vi "Input_Beam_Check_Locations.vi"() -> ()   [LabVIEW 2020]
uses:
  Globals/Constants_global.vi
  Gen Trav/Trav_mode.ctl
  Controls/User_Specific_mode.ctl
  Controls/Tunnel_Coordinates.ctl
  File/Setup_Filetype.ctl
  Globals/LDA_global.vi
panel:
  out "Channel":i32
  out "Setup group":string[][](array[string])
  out "All Beams":bool
  out "BSA IP":string
  out "Unshifted":bool
  out "Laser IP":string
  out "Beam Info":T1(array[cluster])
  in  "Mode":T2(ring)
  out "setups":string[](array[string])
  in  "Traverse Control":T3(array[cluster]) {"Position Change" format="%#.2f"; "Current Position" format="%#.2f"}
  out "Beams to check":string[](array[string])
  out "Error Message":string
  in  "stop":bool
  out "Results":string[][](table)
  out "Working On":string="Green Shifted"
  in  "OK Button":bool
  out "Message":string
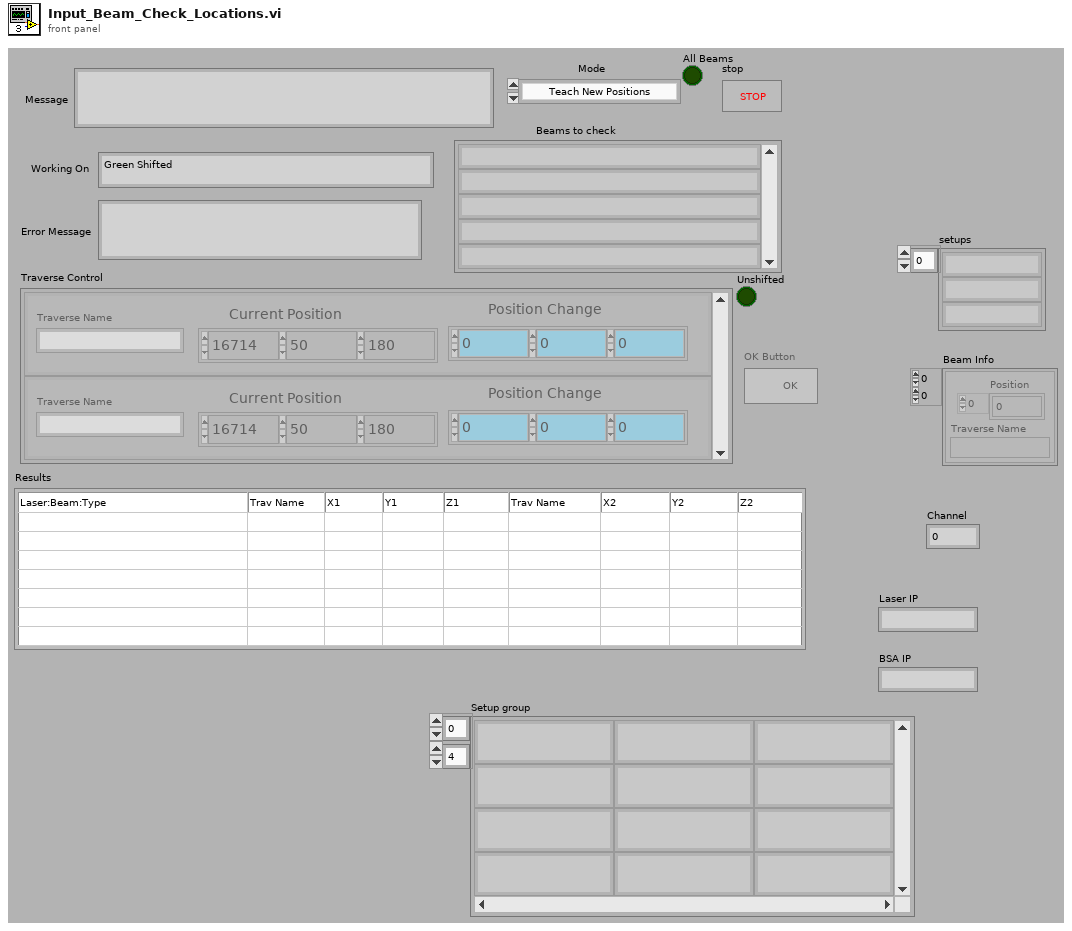
[diagram p1: front panel]
types:
  T1 = cluster{"Position":sgl[], "Traverse Name":string}[][]
  T2 = enum16{"Teach New Positions", "Update Existing Positions"}
  T3 = cluster{"Traverse Name":string, "Current Position":sgl[], "Position Change":sgl[]}[]
  T4 = enum16{"Zero or one", "One", "Zero or more", "One or more"}
  T5 = typedef "Setup_Filetype.ctl" = enum16{"Measurement Setups", "Calibration Setups", "General", "Results File Plotter Setups", "Speed Calib Tweaks"}
  T6 = cluster{"Traverse Name":string, "Current Position":sgl[], "Position Change":sgl[]}
  T7 = typedef "Tunnel_Coordinates.ctl" = enum16{"Work in Tunnel Coordinates", "Work in Model Coordinates"}
  T8 = typedef "User_Specific_mode.ctl" = enum16{"Check VI only", "Run VI"}
  T9 = typedef "Trav_mode.ctl" = enum16{"Move traverse", "Read traverse position", "Teach Position"}
  T10 = enum8{"Enabled", "Disabled", "Disabled and Grayed Out"}
  T11 = typedef "LDA_Channel.ctl" = cluster{"Wavelength (nm)":dbl, "Vel Comp":string, "Max Velocity":dbl, "Min Velocity":dbl, "Max Record length":u16, "Signal gain (dB)":i16, "High voltage":i16, "Optics Conversion Factor":dbl, "Min Record length":u16, "Multiply Velocity by -1":bool, "Signal to Noise Ratio":string, "Validation Ratio":string, "Probe":string, "Laser":string, "BSA":string, "Lense":string, "Beam Separation (mm)":dbl, "Focal Length (mm)":dbl, "COLOUR":u32, "BSA IP":string, "Velocity Range (m/s)":dbl, "Centre Velocity (m/s)":dbl, "Unshifted mW":dbl, "Shifted mW":dbl, "Bandwidth Hz":dbl, "Req Sampling Rate Hz":dbl, "Ch":i32, "CenterFreq Hz":dbl, "Laser IP":string, "Sync Delay (s)":dbl}
  T12 = cluster{"Position":dbl[], "Traverse Name":string}[][]
  T13 = cluster{"Position":dbl[], "Traverse Name":string}
  T14 = cluster{"Position":sgl[], "Traverse Name":string}[]
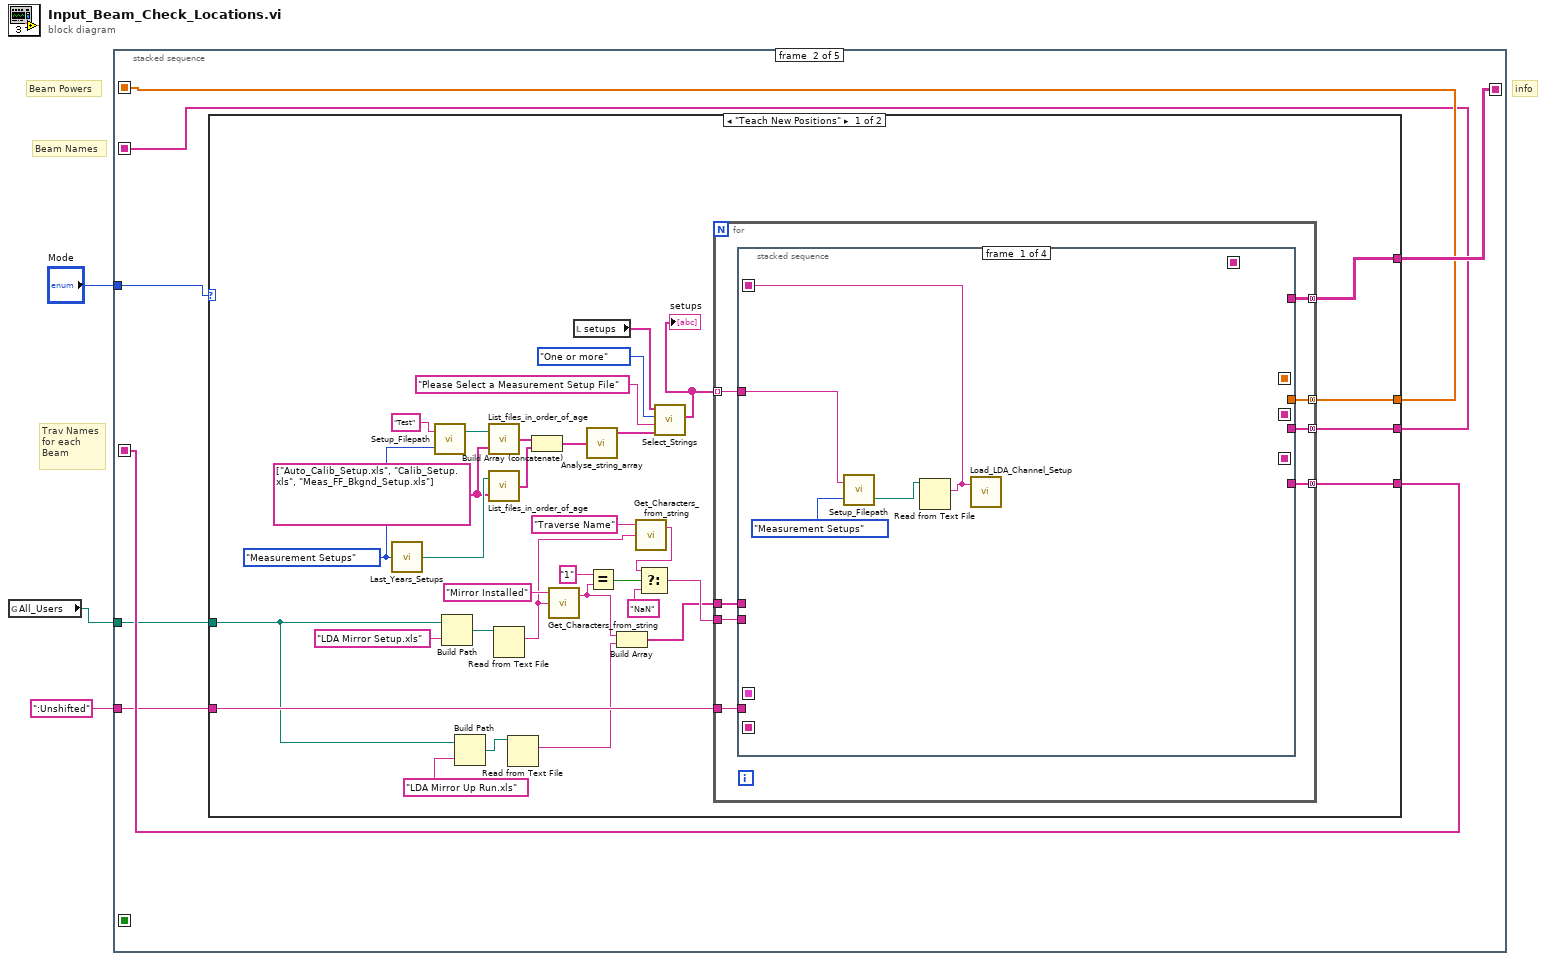
[diagram p0: block diagram]
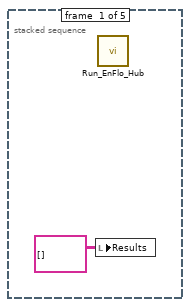
[diagram p2: hidden frame]
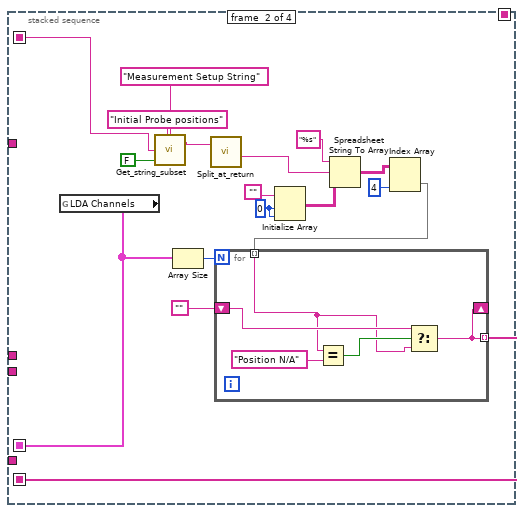
[diagram p3: hidden frame]
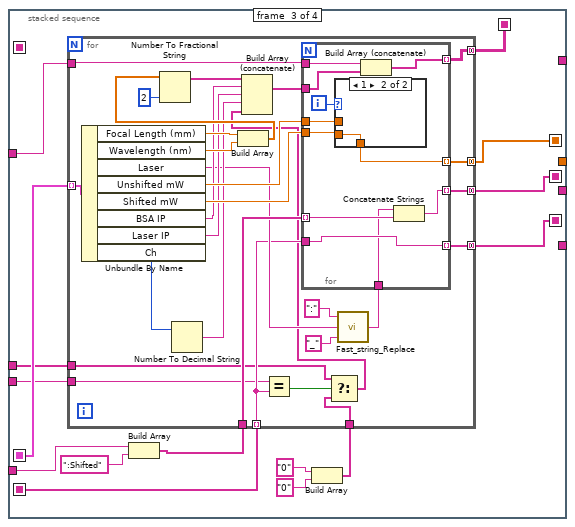
[diagram p4: hidden frame]
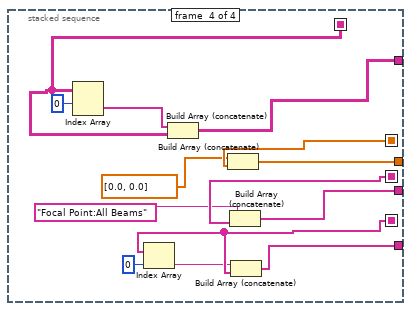
[diagram p6: hidden frame]
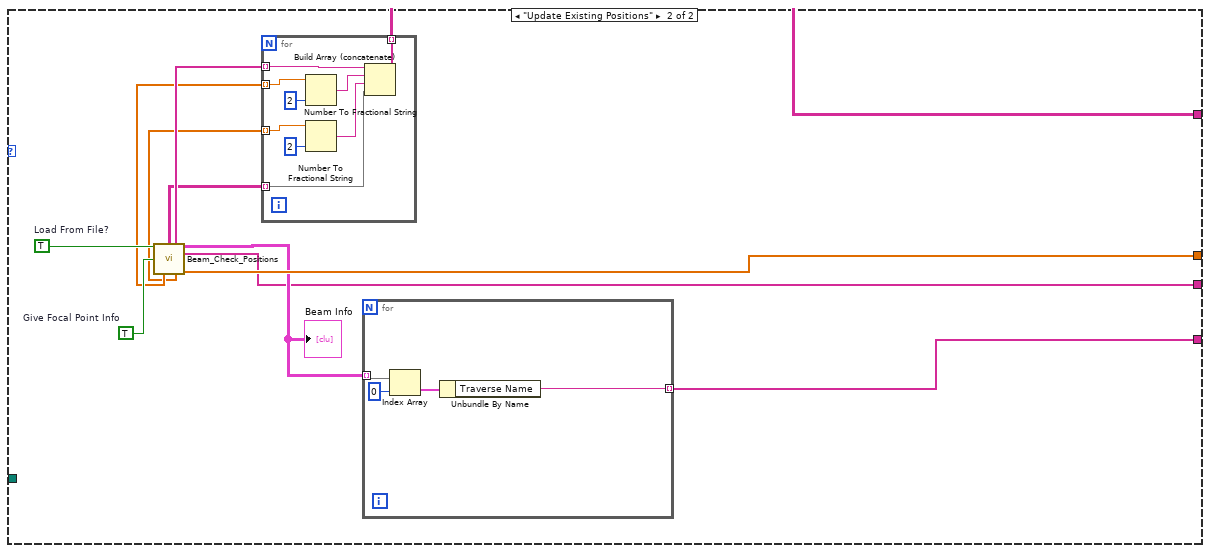
[diagram p7: hidden frame]
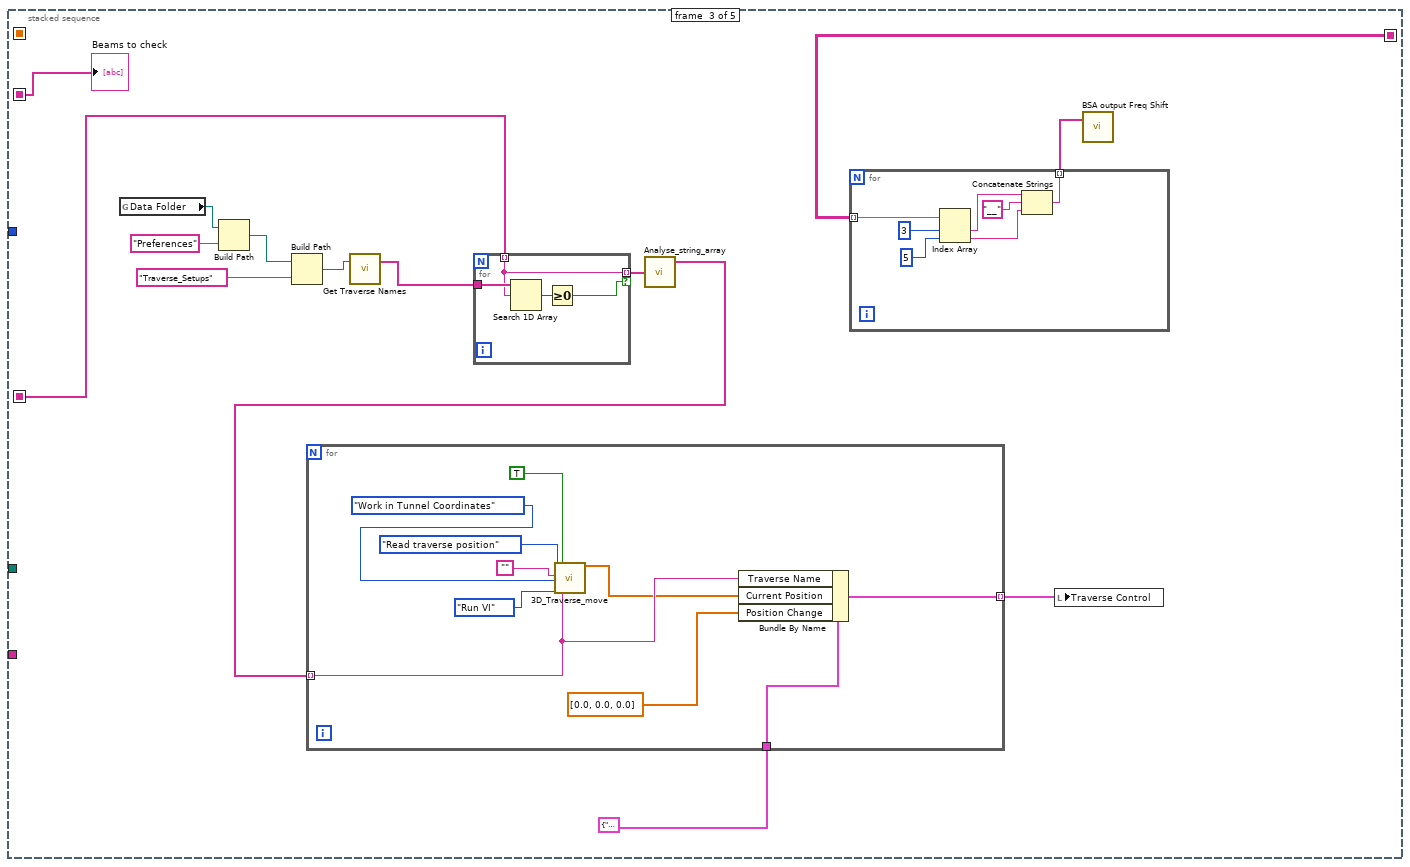
[diagram p8: hidden frame]
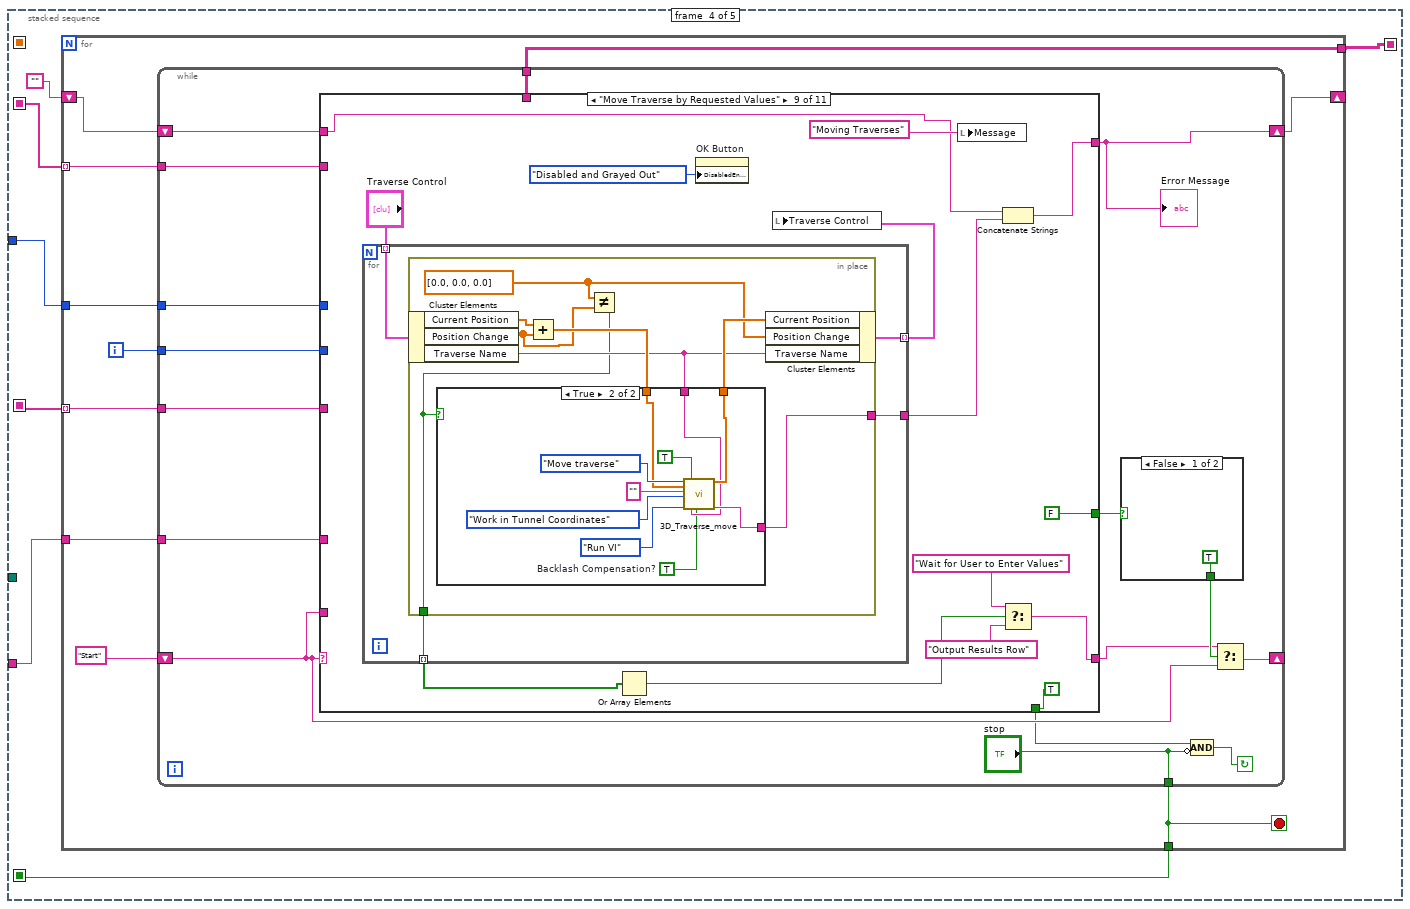
[diagram p9: hidden frame]
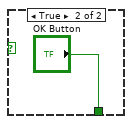
[diagram p10: hidden frame]
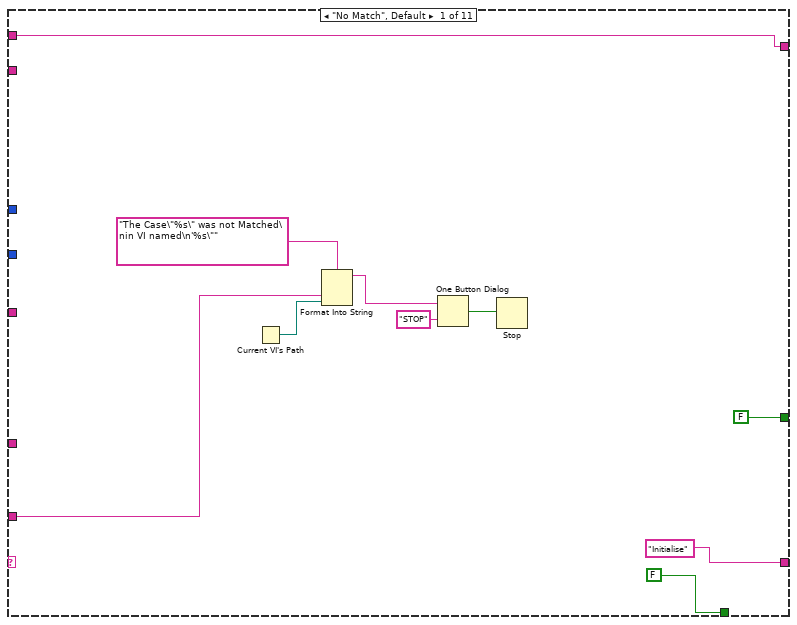
[diagram p11: hidden frame]
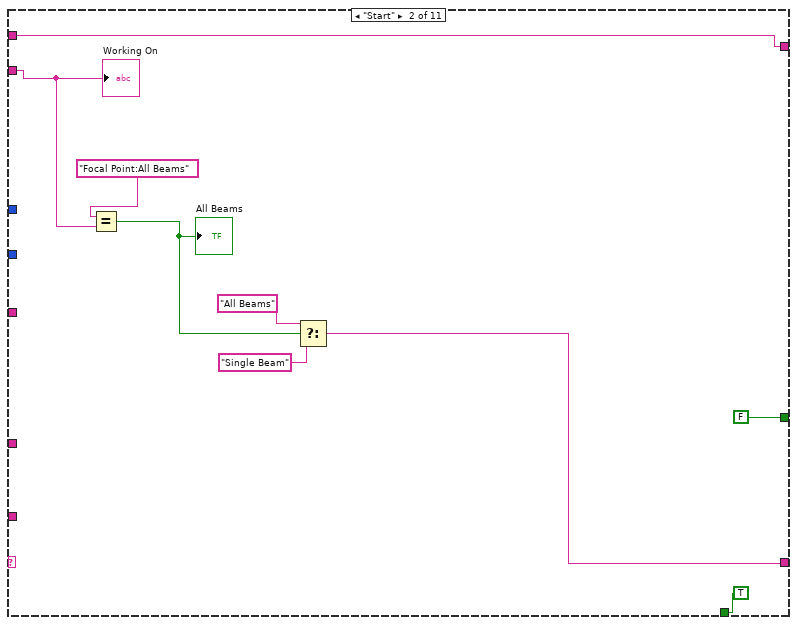
[diagram p12: hidden frame]
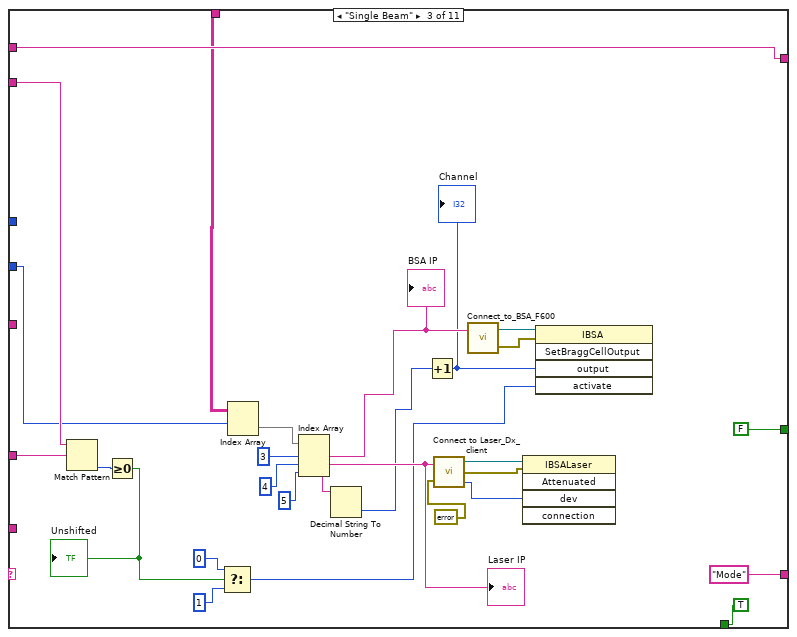
[diagram p13: hidden frame]
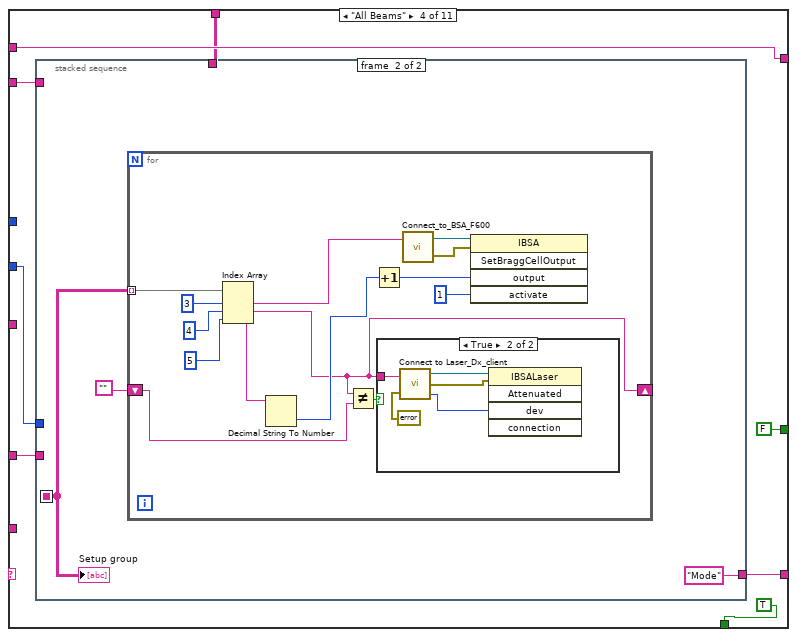
[diagram p14: hidden frame]
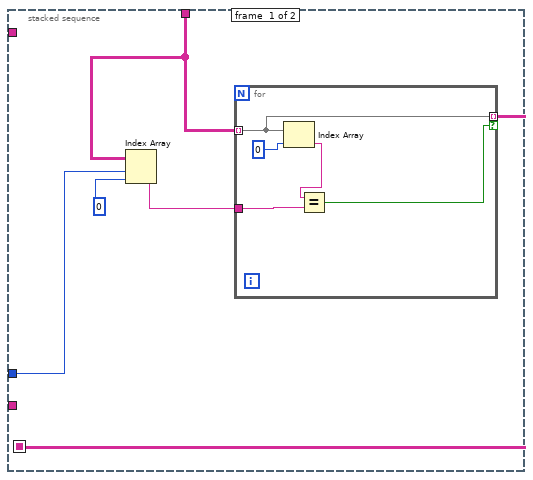
[diagram p15: hidden frame]
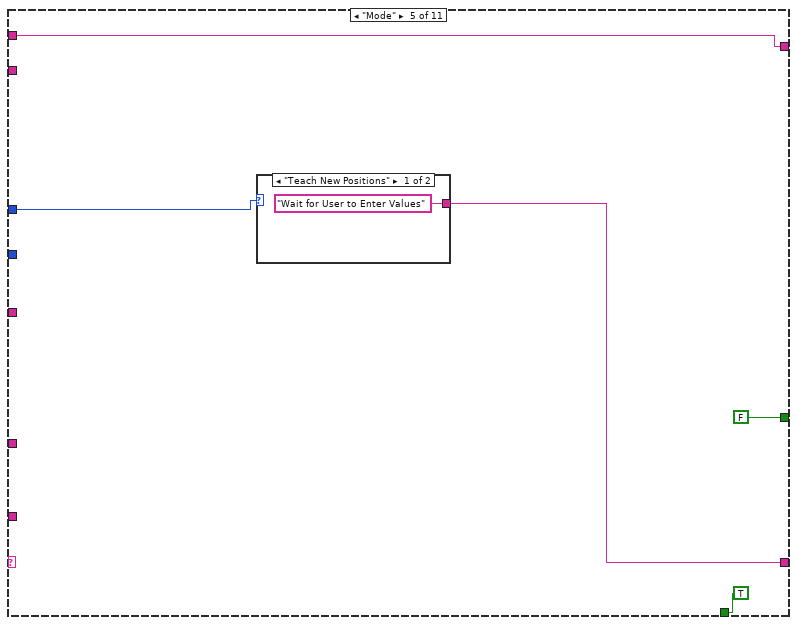
[diagram p17: hidden frame]
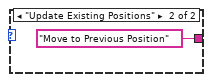
[diagram p18: hidden frame]
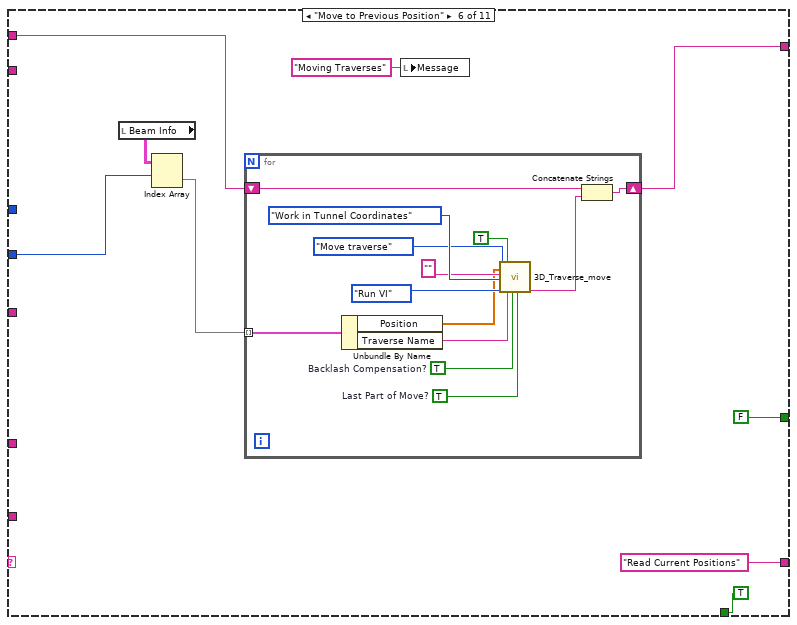
[diagram p19: hidden frame]
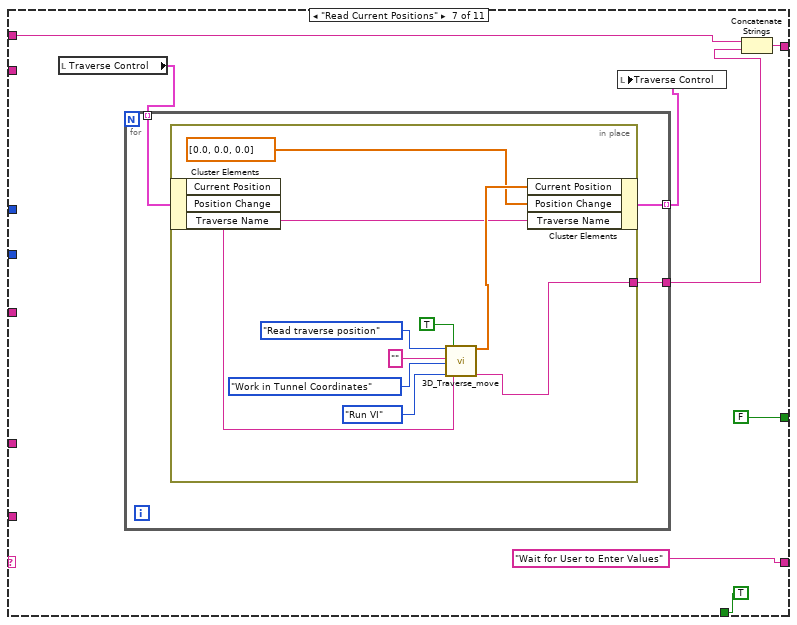
[diagram p20: hidden frame]
diagram:
  # "Beam Powers"
  # "info"
  # "Trav Names\nfor each\nBeam"
  # "Beam Names"
  n1 = global read "Constants_global.vi" "All_Users"() -> (w1:path)
  n2 = stacked-sequence {
    seq-local: [_ w11 _ _ _] -> [_ _ w182 w214 _]
    seq-local: [_ w8 _ _ _] -> [_ _ w179 w216 _]
    seq-local: [_ w10 _ _ _] -> [_ _ w178 w210 w494]
    seq-local: [_ w9 _ _ _] -> [_ _ _ _ w492]
    seq-local: [_ _ _ w213 _] -> [_ _ _ _ w493]
    tunnel: "Mode" -> [_ w7 _ w212 _]
    tunnel: ":Unshifted" ("f") -> [_ w6 _ w211 _]
    tunnel: w1 -> [_ w5 _ _ _]
    frame #0 {
      n3 = local write "Results"(string[][] [] ("Results")) -> ()
      n4 = call "Run_EnFlo_Hub.vi"() -> ()  [unwired: 7 in, 1 out]
    }
    frame #1 {
      n5 = case shown="\"Teach New Positions\"" w7 {
        tunnel: [w33 w158] -> w11
        tunnel: [w32 w155] -> w10
        tunnel: [w31 w160] -> w9
        tunnel: [w30 w157] -> w8
        tunnel: w6 -> [w28 _]
        tunnel: w5 -> [w22 _]
        frame "Teach New Positions" {
          w40 = string[] ["Auto_Calib_Setup.xls", "Calib_Setup.xls", "Meas_FF_Bkgnd_Setup.xls"] ("file names")
          w39 = Setup_Filetype."Measurement Setups" ("Setup File Type")
          n6 = call "Last_Years_Setups.vi"("Setup File Type"=w39) -> ("Directory"=w41:path)
          n7 = call "Setup_Filepath.vi"("Setup File Type"=w39, "Filename in"="Test") -> ("Directory"=w44:path)  [unwired: 1 out]
          n8 = Build Path(base path=w22, name or relative path="LDA Mirror Setup.xls") -> (appended path=w25:path)
          n9 = Build Path(base path=w22, name or relative path="LDA Mirror Up Run.xls") -> (appended path=w23:path)
          n10 = call "List_files_in_order_of_age.vi"("Files to Hide"=w40, "Folder"=w44) -> ("file names"=w38:string[])
          n11 = call "List_files_in_order_of_age.vi"("Files to Hide"=w40, "Folder"=w41) -> ("file names"=w37:string[])
          n12 = Read from Text File(file (use dialog)=w25) -> (text=w17:string)  [unwired: 3 in, 3 out]
          n13 = Read from Text File(file (use dialog)=w23) -> (text=w21:string)  [unwired: 3 in, 3 out]
          n14 = Build Array (concatenate)(w38, w37) -> (w36:string[])
          n15 = call "Get_Characters_from_string.vi"("Input string"=w17, "Variable name"="Mirror Installed") -> ("Value"=w19:string)  [unwired: 1 in, 1 out]
          n16 = local read "setups"() -> (w34:string[])
          n17 = call "Analyse_string_array.vi"("String array"=w36) -> ("Unique strings"=w35:string[])  [unwired: 1 in, 1 out]
          n18 = Equal?(x="1", y=w19) -> (x = y?=w16:bool)
          n19 = Build Array(w19, w21) -> (w12:string[])
          n20 = call "Get_Characters_from_string.vi"("Input string"=w17, "Variable name"="Traverse Name") -> ("Value"=w15:string)  [unwired: 1 in, 1 out]
          n21 = Select(t=w15, s=w16, f="NaN") -> (s? t:f=w13:string)
          n22 = call "Select_Strings.vi"("Available Ch names"=w35, "Message"="Please Select a Measurement Setup File", "Selector mode"=T4."One or more", "Desired Ch names (in)"=w34) -> ("Selected Channel Names"=w29:string[])  [unwired: 2 in, 2 out]
          "setups" <- w29
          n23 = for {
            tunnel: w29 -> [w53] mode=indexing
            tunnel: [w52] -> w30 mode=concatenating
            tunnel: [w51] -> w33 mode=concatenating
            tunnel: [w50] -> w32 mode=concatenating
            tunnel: [w49] -> w31 mode=concatenating
            tunnel: w28 -> [w48]
            tunnel: w13 -> [w47]
            tunnel: w12 -> [w46]
            n24 = stacked-sequence {
              seq-local: [w55 _ _ _] -> [_ w63 _ _]
              seq-local: [_ w60 _ _] -> [_ _ w92 _]
              seq-local: [_ w59 _ _] -> [_ _ w91 _]
              seq-local: [_ _ w89 _] -> [_ _ _ w150]
              seq-local: [_ _ w88 _] -> [_ _ _ w148]
              seq-local: [_ _ w87 _] -> [_ _ _ w146]
              seq-local: [_ _ w86 _] -> [_ _ _ w144]
              tunnel: w53 -> [w54 _ w90 _]
              tunnel: [_ _ _ w145] -> w52
              tunnel: [_ _ _ w143] -> w51
              tunnel: [_ _ _ w149] -> w50
              tunnel: [_ _ _ w147] -> w49
              tunnel: w48 -> [_ _ w85 _]
              tunnel: w47 -> [_ _ w84 _]
              tunnel: w46 -> [_ _ w80 _]
              frame #0 {
                n25 = call "Setup_Filepath.vi"("Setup File Type"=Setup_Filetype."Measurement Setups", "Filename in"=w54) -> ("Filename Out"=w56:path)  [unwired: 1 out]
                n26 = Read from Text File(file (use dialog)=w56) -> (text=w55:string)  [unwired: 3 in, 3 out]
                n27 = call "Load_LDA_Channel_Setup.vi"("Setup file string"=w55) -> ()  [unwired: 2 in]
              }
              frame #1 {
                w72 = 0 ("Dimension Size")
                n28 = global read "LDA_global.vi" "LDA Channels"() -> (w60:T11[])
                n29 = call "Get_string_subset.vi"("String Name"="Measurement Setup String", "Show Dialog?"=FALSE, "String to split"=w63, "File Label"="Initial Probe positions") -> ("Output string"=w74:string)  [unwired: 1 out]
                n30 = Array Size(array=w60) -> (size(s)=w61:i32)
                n31 = call "Split_at_return.vi"("String"=w74) -> ("after substring"=w69:string)  [unwired: 1 in, 3 out]
                n32 = Initialize Array("", w72, w72) -> (w73:string[][])
                n33 = Spreadsheet String To Array(format string="%s", spreadsheet string=w69, array type (2D Dbl)=w73) -> (array=w65:string[][])  [unwired: 1 out]
                n34 = Index Array(array=w65, index (col)=4 ("disabled index (col)")) -> (element=w62:string[])  [unwired: 1 in]
                n35 = for {
                  N: w61 -> [_]
                  tunnel: w62 -> [w76] mode=indexing
                  shift-right: [w75] -> _
                  shift-left: "" -> [w77]
                  tunnel: [w75] -> w59 mode=indexing
                  n36 = Equal?(x=w76, y="Position N/A") -> (x = y?=w78:bool)
                  n37 = Select(t=w77, s=w78, f=w76) -> (s? t:f=w75:string)
                }
              }
              frame #2 {
                n38 = Build Array(w85, ":Shifted") -> (w93:string[])
                n39 = Build Array("0", "0") -> (w81:string[])
                n40 = for {
                  tunnel: w92 -> [w123] mode=indexing
                  tunnel: w93 -> [w122]
                  tunnel: [w121] -> w87 mode=concatenating
                  tunnel: w91 -> [w100] mode=indexing
                  tunnel: [w120] -> w86 mode=concatenating
                  tunnel: [w117] -> w88 mode=concatenating
                  tunnel: [w116] -> w89 mode=concatenating
                  tunnel: w90 -> [w115]
                  tunnel: w84 -> [w99]
                  tunnel: w81 -> [w97]
                  tunnel: w80 -> [w96]
                  n41 = Unbundle By Name(w123) -> ("Focal Length (mm)"=w112:dbl, "Wavelength (nm)"=w113:dbl, "Laser"=w104:string, "Unshifted mW"=w119:dbl, "Shifted mW"=w118:dbl, "BSA IP"=w108:string, "Laser IP"=w107:string, "Ch"=w106:i32)
                  n42 = Number To Decimal String(number=w106) -> (decimal integer string=w105:string)  [unwired: 1 in]
                  n43 = Build Array(w112, w113) -> (w111:dbl[])
                  n44 = Number To Fractional String(number=w111, precision (6)=i16 2) -> (F-format string=w110:string[])  [unwired: 2 in]
                  n45 = Equal?(x=w99, y=w100) -> (x = y?=w98:bool)
                  n46 = Select(t=w96, s=w98, f=w97) -> (s? t:f=w95:string[])
                  n47 = Build Array (concatenate)(w110, w108, w107, w105, w95) -> (w109:string[])
                  n48 = call "Fast_string_Replace.vi"("Replace match with:"="_", "Input String"=w104, "regular expression"=":") -> ("Output String"=w101:string)  [unwired: 1 in, 1 out]
                  n49 = for {
                    tunnel: w122 -> [w134] mode=indexing
                    tunnel: [w131] -> w121 mode=indexing
                    tunnel: w100 -> [w128]
                    tunnel: [w128] -> w120 mode=indexing
                    tunnel: w119 -> [w132]
                    tunnel: w118 -> [w130]
                    tunnel: [w129] -> w117 mode=indexing
                    tunnel: [w125] -> w116 mode=indexing
                    tunnel: w115 -> [w127]
                    tunnel: w109 -> [w126]
                    tunnel: w101 -> [w124]
                    i -> [w133]
                    n50 = case shown="1" w133 {
                      tunnel: [w135 w136] -> w129
                      tunnel: w132 -> [w135 _]
                      tunnel: w130 -> [_ w136]
                      frame 0, Default {
                      }
                      frame 1 {
                      }
                    }
                    n51 = Build Array (concatenate)(w127, w126) -> (w125:string[])
                    n52 = Concatenate Strings(w124, w134) -> (w131:string)
                  }
                }
              }
              frame #3 {
                n53 = Index Array(array=w150, index (row)=0) -> (element=w141:string[])  [unwired: 1 in]
                n54 = Index Array(array=w144, index=0 ("index (row)")) -> (element=w137:string)
                n55 = Build Array (concatenate)(w141, w150) -> (w149:string[][])
                n56 = Build Array (concatenate)(dbl[] [0.0, 0.0], w148) -> (w147:dbl[])
                n57 = Build Array (concatenate)("Focal Point:All Beams", w146) -> (w145:string[])
                n58 = Build Array (concatenate)(w137, w144) -> (w143:string[])
              }
            }
          }
        }
        frame "Update Existing Positions" {
          w154 = TRUE  # Give Focal Point Info
          w161 = TRUE  # Load From File?
          n59 = call "Beam_Check_Positions.vi"("Load From File?"=w161, "Give Focal Point Info (F)"=w154) -> ("More Info"=w151:string[][], "Setup File"=w156:string[], "Beam Info"=w159:T12, "Beam Names"=w157:string[], "Focal Length"=w153:dbl[], "Wavelength (nm)"=w152:dbl[], "Power (mW)"=w160:dbl[])  [unwired: 5 in, 2 out]
          "Beam Info" <- w159
          n60 = for {
            tunnel: w156 -> [w170] mode=indexing
            tunnel: w153 -> [w169] mode=indexing
            tunnel: [w167] -> w155 mode=indexing
            tunnel: w152 -> [w166] mode=indexing
            tunnel: w151 -> [w162] mode=indexing
            n61 = Number To Fractional String(number=w169, precision (6)=i16 2) -> (F-format string=w168:string)  [unwired: 2 in]
            n62 = Number To Fractional String(number=w166, precision (6)=i16 2) -> (F-format string=w165:string)  [unwired: 2 in]
            n63 = Build Array (concatenate)(w170, w168, w165, w162) -> (w167:string[])
          }
          n64 = for {
            tunnel: w159 -> [w174] mode=indexing
            tunnel: [w171] -> w158 mode=indexing
            n65 = Index Array(array=w174, index=0) -> (element=w172:T13)
            n66 = Unbundle By Name(w172) -> ("Traverse Name"=w171:string)
          }
        }
      }
    }
    frame #2 {
      n67 = global read "Constants_global.vi" "Data Folder"() -> (w188:path)
      n68 = Build Path(base path=w188, name or relative path="Preferences") -> (appended path=w187:path)
      n69 = Build Path(base path=w187, name or relative path="Traverse_Setups") -> (appended path=w176:path)
      n70 = call "Get Traverse Names.vi"("Traverse\nSetup\nFolder"=w176) -> ("Traverse Names"=w175:string[])  [unwired: 1 in, 1 out]
      n71 = for {
        tunnel: w175 -> [w209]
        tunnel: w182 -> [w207] mode=indexing
        tunnel: [w207] -> w181 mode=indexing if=w206
        n72 = Search 1D Array(1D array=w209, element=w207) -> (index of element=w208:i32)  [unwired: 1 in]
        n73 = Greater Or Equal To 0?(x=w208) -> (x >= 0?=w206:bool)
      }
      n74 = call "Analyse_string_array.vi"("String array"=w181) -> ("Unique strings"=w180:string[])  [unwired: 1 in, 1 out]
      n75 = for {
        tunnel: w180 -> [w202] mode=indexing
        tunnel: T6 {"Traverse Name"="", "Current Position"=[], "Position Change"=[]} ("Cluster 2") -> [w203]
        tunnel: [w198] -> w183 mode=indexing
        n76 = call "3D_Traverse_move.vi"("Mode"=Trav_mode."Read traverse position", "Extra command String"="", "Work in Tunnel Coordinates"=Tunnel_Coordinates."Work in Tunnel Coordinates", "Simulate/Run"=User_Specific_mode."Run VI", "Route Checking?"=TRUE, "Traverse name"=w202) -> ("Trav Position achieved"=w200:sgl[])  [unwired: 10 in, 3 out]
        n77 = Bundle By Name(cluster=w203, "Traverse Name"=w202, "Current Position"=w200, "Position Change"=sgl[] [0.0, 0.0, 0.0]) -> (w198:T6)
      }
      n78 = for {
        tunnel: w178 -> [w193] mode=indexing
        tunnel: [w191] -> w177 mode=indexing
        n79 = Index Array(array=w193, index #1=3 ("index"), index #2=5 ("index")) -> (element #1=w192:string, element #2=w189:string)
        n80 = Concatenate Strings(w192, "__" ("string"), w189) -> (w191:string)
      }
      n81 = local write "Traverse Control"(w183) -> ()
      n82 = call "BSA output Freq Shift.vi"("BSAIP__ChNum"=w177) -> ()  [unwired: 2 in, 1 out]
      "Beams to check" <- w179
    }
    frame #3 {
      n83 = for {
        tunnel: w216 -> [w225] mode=indexing
        shift-right: [w223] -> _
        shift-left: "" -> [w224]
        tunnel: w214 -> [w222] mode=indexing
        tunnel: [w221] -> w213
        tunnel: w212 -> [w220]
        tunnel: w211 -> [w218]
        tunnel: w210 -> [w217]
        i -> [w219]
        stop <- w221 stop-if-true
        n84 = while {
          shift-left: "Start" -> [w240]
          shift-right: [w239] -> _
          shift-right: [w235] -> w223
          shift-left: w224 -> [w234]
          tunnel: w225 -> [w233]
          tunnel: w222 -> [w232]
          tunnel: ["stop"] -> w221
          tunnel: w220 -> [w230]
          tunnel: w219 -> [w229]
          tunnel: w218 -> [w228]
          tunnel: w217 -> [w227]
          stop <- w236 continue-if-true
          n85 = case shown="\"Move Traverse by Requested Values\"" w240 {
            tunnel: [FALSE TRUE TRUE TRUE TRUE TRUE TRUE TRUE TRUE TRUE FALSE] -> w237
            tunnel: ["Initialise" w259 "Mode" ("t") w292 w335 "Read Current Positions" ("t") "Wait for User to Enter Values" ("f") "Move Traverse by Requested Values" w400 "End" ("t") "End" ("t")] -> w241
            tunnel: w240 -> [w249 _ _ _ _ _ _ _ _ _ _]
            tunnel: [FALSE FALSE FALSE FALSE FALSE FALSE FALSE TRUE FALSE FALSE FALSE] -> w238
            tunnel: [w245 w256 w289 w297 w332 w342 w365 w383 w397 w434 w457] -> w235
            tunnel: w234 -> [w245 w256 w289 w297 w332 w343 w363 w383 w396 w434 w457]
            tunnel: w233 -> [_ w262 w286 w295 _ _ _ _ _ _ _]
            tunnel: w232 -> [_ _ _ _ _ _ _ _ _ w430 _]
            tunnel: w230 -> [_ _ _ _ w336 _ _ _ _ _ _]
            tunnel: w229 -> [_ _ w284 w293 _ w345 _ _ _ _ _]
            tunnel: w228 -> [_ _ w288 w296 _ _ _ _ _ _ _]
            tunnel: w227 -> [_ _ w285 w294 _ _ _ _ _ _ _]
            frame "No Match", Default {
              n86 = Current VI's Path() -> (path=w248:path)
              n87 = Format Into String(format string="The Case\"%s\" was not Matched\nin VI named\n'%s\"" ("Format String"), w249, w248) -> (resulting string=w252:string)  [unwired: 2 in, 1 out]
              n88 = One Button Dialog(message=w252, button name ("OK")="STOP") -> (true=w250:bool)
              n89 = Stop(stop? (T)=w250) -> ()
            }
            frame "Start" {
              n90 = Equal?(x="Focal Point:All Beams", y=w262) -> (x = y?=w261:bool)
              "All Beams" <- w261
              n91 = Select(t="All Beams", s=w261, f="Single Beam") -> (s? t:f=w259:string)
              "Working On" <- w262
            }
            frame "Single Beam" {
              n92 = Match Pattern(string=w286, regular expression=w288) -> (offset past match=w287:i32)  [unwired: 1 in, 3 out]
              n93 = Greater Or Equal To 0?(x=w287) -> (x >= 0?=w276:bool)
              "Unshifted" <- w276
              n94 = Select(t=0 ("SetBraggCellOutputFreq"), s=w276, f=1 ("SetBraggCellOutputFreq")) -> (s? t:f=w273:i32)
              n95 = Index Array(array=w285, index (row)=w284) -> (element=w270:string[])  [unwired: 1 in]
              n96 = Index Array(array=w270, index #1=3 ("index"), index #2=4 ("index"), index #3=5 ("index")) -> (element #1=w277:string, element #2=w283:string, element #3=w266:string)
              "Laser IP" <- w283
              "BSA IP" <- w277
              n97 = Decimal String To Number(string=w266) -> (number=w272:i32)  [unwired: 2 in, 1 out]
              n98 = Increment(x=w272) -> (x+1=w265:i32)
              "Channel" <- w265
              n99 = call "Connect to Laser_Dx_client.vi"("Laser IP Number"=w283, "error in (no error)"=errorcluster {"status"=FALSE, "code"=0, "source"=""}) -> ("Laser_Dx"=w282:refnum<k7>, "error out"=w281:errorcluster, "Channel"=w280:i64)
              n100 = call "Connect_to_BSA_F600.vi"("BSA IP Number"=w277) -> ("error out"=w278:errorcluster, "F600"=w279:refnum<k7>)  [unwired: 1 in]
              n101 = invoke class="IBSALaser" method="Attenuated"(reference=w282, error in=w281, "dev"=w280) -> ()  [unwired: 2 in, 5 out]
              n102 = invoke class="IBSA" method="SetBraggCellOutput"(reference=w279, error in=w278, "output"=w265, "activate"=w273) -> ()  [unwired: 1 in, 5 out]
            }
            frame "All Beams" {
              n103 = stacked-sequence {
                seq-local: [w300 _] -> [_ w311]
                tunnel: w296 -> [_ _]
                tunnel: w295 -> [_ _]
                tunnel: w294 -> [w301 _]
                tunnel: w293 -> [w304 _]
                tunnel: [_ "Mode" ("t")] -> w292
                frame #0 {
                  n104 = Index Array(array=w301, index (row)=w304, index (col)=0 ("disabled index (col)")) -> (element=w302:string)
                  n105 = for {
                    tunnel: w302 -> [w309]
                    tunnel: w301 -> [w306] mode=indexing
                    tunnel: [w306] -> w300 mode=indexing if=w305
                    n106 = Index Array(array=w306, index=0 ("disabled index (col)")) -> (element=w307:string)
                    n107 = Equal?(x=w307, y=w309) -> (x = y?=w305:bool)
                  }
                }
                frame #1 {
                  n108 = for {
                    shift-right: [w316] -> _
                    shift-left: "" -> [w315]
                    tunnel: w311 -> [w317] mode=indexing
                    n109 = Index Array(array=w317, index #1=3 ("index"), index #2=4 ("index"), index #3=5 ("index")) -> (element #1=w324:string, element #2=w316:string, element #3=w319:string)
                    n110 = Decimal String To Number(string=w319) -> (number=w323:i32)  [unwired: 2 in, 1 out]
                    n111 = Not Equal?(x=w316, y=w315) -> (x != y?=w314:bool)
                    n112 = Increment(x=w323) -> (x+1=w313:i32)
                    n113 = case shown="True" w314 {
                      tunnel: w316 -> [_ w331]
                      frame False {
                      }
                      frame True {
                        n114 = call "Connect to Laser_Dx_client.vi"("Laser IP Number"=w331, "error in (no error)"=errorcluster {"status"=FALSE, "code"=0, "source"=""}) -> ("Laser_Dx"=w330:refnum<k7>, "error out"=w329:errorcluster, "Channel"=w328:i64)
                        n115 = invoke class="IBSALaser" method="Attenuated"(reference=w330, error in=w329, "dev"=w328) -> ()  [unwired: 2 in, 5 out]
                      }
                    }
                    n116 = call "Connect_to_BSA_F600.vi"("BSA IP Number"=w324) -> ("error out"=w325:errorcluster, "F600"=w326:refnum<k7>)  [unwired: 1 in]
                    n117 = invoke class="IBSA" method="SetBraggCellOutput"(reference=w326, error in=w325, "output"=w313, "activate"=1 ("SetBraggCellOutputFreq")) -> ()  [unwired: 1 in, 5 out]
                  }
                  "Setup group" <- w311
                }
              }
            }
            frame "Mode" {
              n118 = case shown="\"Teach New Positions\"" w336 {
                tunnel: ["Wait for User to Enter Values" ("f") "Move to Previous Position"] -> w335
                frame "Teach New Positions" {
                }
                frame "Update Existing Positions" {
                }
              }
            }
            frame "Move to Previous Position" {
              n119 = local read "Beam Info"() -> (w347:T1)
              n120 = Index Array(array=w347, index (row)=w345) -> (element=w346:T14)  [unwired: 1 in]
              n121 = for {
                shift-right: [w353] -> w342
                shift-left: w343 -> [w352]
                tunnel: w346 -> [w350] mode=indexing
                w348 = TRUE  # Last Part of Move?
                w349 = TRUE  # Backlash Compensation?
                n122 = Unbundle By Name(w350) -> ("Position"=w355:sgl[], "Traverse Name"=w354:string)
                n123 = call "3D_Traverse_move.vi"("Mode"=Trav_mode."Move traverse", "Position"=w355, "Extra command String"="", "Work in Tunnel Coordinates"=Tunnel_Coordinates."Work in Tunnel Coordinates", "Simulate/Run"=User_Specific_mode."Run VI", "Route Checking?"=TRUE, "Traverse name"=w354, "Backlash Compensation?"=w349, "Last Part of Move?"=w348) -> ("Error String"=w351:string)  [unwired: 7 in, 3 out]
                n124 = Concatenate Strings(w352, w351) -> (w353:string)
              }
              n125 = local write "Message"("Moving Traverses" ("Message")) -> ()
            }
            frame "Read Current Positions" {
              n126 = local read "Traverse Control"() -> (w368:T3)
              n127 = for {
                tunnel: [w371] -> w364
                tunnel: w368 -> [w370] mode=indexing
                tunnel: [w369] -> w366 mode=indexing
                n128 = in-place {
                  in-place-border: [w380] -> w371
                  n129 = in-place-cluster #1(w370) -> ("Traverse Name"=w377:string)  [unwired: 2 out]
                  n130 = call "3D_Traverse_move.vi"("Mode"=Trav_mode."Read traverse position", "Extra command String"="", "Work in Tunnel Coordinates"=Tunnel_Coordinates."Work in Tunnel Coordinates", "Simulate/Run"=User_Specific_mode."Run VI", "Route Checking?"=TRUE, "Traverse name"=w377) -> ("Trav Position achieved"=w379:sgl[], "Error String"=w380:string)  [unwired: 10 in, 2 out]
                  n131 = in-place-cluster #1("Current Position"=w379, "Position Change"=sgl[] [0.0, 0.0, 0.0] ("Green Position Change"), "Traverse Name"=w377) -> (w369:T6)
                }
              }
              n132 = local write "Traverse Control"(w366) -> ()
              n133 = Concatenate Strings(w363, w364) -> (w365:string)
            }
            frame "Wait for User to Enter Values" {
              n134 = local read "Working On"() -> (w384:string)
              n135 = property on="OK Button" class="Bool"("DisabledEnum"=T10."Enabled" ("Disabled")) -> ()  [unwired: 2 in, 2 out]
              n136 = Format Into String(format string="Please get the %s beam into the power meter by editing Positions then Press OK", w384) -> (resulting string=→"Message":string)  [unwired: 2 in, 1 out]
            }
            frame "Move Traverse by Requested Values" {
              n137 = for {
                tunnel: [w406] -> w398
                tunnel: "Traverse Control" -> [w405] mode=indexing
                tunnel: [w404] -> w394 mode=indexing
                tunnel: [w403] -> w391 mode=indexing
                n138 = in-place {
                  in-place-border: [w414] -> w406
                  in-place-border: [w407] -> w404
                  w409 = sgl[] [0.0, 0.0, 0.0] ("Green Position Change")
                  n139 = in-place-cluster #2(w405) -> ("Current Position"=w413:sgl[], "Position Change"=w410:sgl[], "Traverse Name"=w408:string)
                  n140 = Add(x=w413, y=w410) -> (x+y=w412:sgl[])
                  n141 = Not Equal?(x=w409, y=w410) -> (x != y?=w407:bool)
                  n142 = case shown="True" w407 {
                    tunnel: ["" w426] -> w414
                    tunnel: w412 -> [w416 w420]
                    tunnel: [w416 w419] -> w411
                    tunnel: w408 -> [_ w418]
                    frame False {
                    }
                    frame True {
                      w417 = TRUE  # Backlash Compensation?
                      n143 = call "3D_Traverse_move.vi"("Mode"=Trav_mode."Move traverse", "Position"=w420, "Extra command String"="", "Work in Tunnel Coordinates"=Tunnel_Coordinates."Work in Tunnel Coordinates", "Simulate/Run"=User_Specific_mode."Run VI", "Route Checking?"=TRUE, "Traverse name"=w418, "Backlash Compensation?"=w417) -> ("Trav Position achieved"=w419:sgl[], "Error String"=w426:string)  [unwired: 8 in, 2 out]
                    }
                  }
                  n144 = in-place-cluster #2("Current Position"=w411, "Position Change"=w409, "Traverse Name"=w408) -> (w403:T6)
                }
              }
              n145 = Or Array Elements(Boolean array=w394) -> (logical OR=w393:bool)
              n146 = property on="OK Button" class="Bool"("DisabledEnum"=T10."Disabled and Grayed Out" ("Disabled")) -> ()  [unwired: 2 in, 2 out]
              n147 = local write "Traverse Control"(w391) -> ()
              n148 = local write "Message"("Moving Traverses") -> ()
              n149 = Concatenate Strings(w396, w398) -> (w397:string)
              n150 = Select(t="Wait for User to Enter Values" ("f"), s=w393, f="Output Results Row" ("t")) -> (s? t:f=w400:string)
            }
            frame "Output Results Row" {
              n151 = local read "Traverse Control"() -> (w429:T3)
              n152 = for {
                tunnel: w429 -> [w449] mode=indexing
                tunnel: [w448] -> w431 mode=indexing
                n153 = Unbundle By Name(w449) -> ("Traverse Name"=w448:string)
              }
              n154 = local read "Working On"() -> (w438:string)
              n155 = Search 1D Array(1D array=w431, element=w430) -> (index of element=w427:i32)  [unwired: 1 in]
              n156 = case shown="Default" w427 {
                selector: w427 -> [w441 _]
                tunnel: w429 -> [w445 w447]
                tunnel: [w442 w447] -> w428
                frame Default {
                  n157 = Delete From Array(array=w445, length=1, index=w441) -> (array with subset deleted=w443:T3)  [unwired: 1 out]
                  n158 = Index Array(array=w445, index=w441) -> (element=w444:T6)
                  n159 = Build Array (concatenate)(w444, w443) -> (w442:T3)
                }
                frame -1 {
                }
              }
              n160 = for {
                tunnel: w428 -> [w455] mode=indexing
                tunnel: [w450] -> w432 mode=concatenating
                n161 = Unbundle By Name(w455) -> ("Traverse Name"=w451:string, "Current Position"=w453:sgl[])
                n162 = Number To Fractional String(number=w453, precision (6)=i16 2) -> (F-format string=w452:string[])  [unwired: 2 in]
                n163 = Build Array (concatenate)(w451, w452) -> (w450:string[])
              }
              n164 = Build Array (concatenate)(w438, w432) -> (w436:string[])
              n165 = local read "Results"() -> (w437:string[][])
              n166 = Build Array (concatenate)(w437, w436) -> (→"Results":string[][])
            }
            frame "End" {
              n167 = local read "All Beams"() -> (w456:bool)
              n168 = case shown="True" w456 {
                frame False {
                  n169 = local read "Laser IP"() -> (w466:string)
                  n170 = local read "BSA IP"() -> (w467:string)
                  n171 = local read "Channel"() -> (w462:i32)
                  n172 = call "Connect to Laser_Dx_client.vi"("Laser IP Number"=w466, "error in (no error)"=errorcluster {"status"=FALSE, "code"=0, "source"=""}) -> ("Laser_Dx"=w465:refnum<k7>, "error out"=w464:errorcluster, "Channel"=w463:i64)
                  n173 = call "Connect_to_BSA_F600.vi"("BSA IP Number"=w467) -> ("error out"=w469:errorcluster, "F600"=w470:refnum<k7>)  [unwired: 1 in]
                  n174 = invoke class="IBSA" method="SetBraggCellOutput"(reference=w470, error in=w469, "output"=w462, "activate"=0 ("output")) -> ()  [unwired: 1 in, 5 out]
                  n175 = invoke class="IBSALaser" method="ShutterClosed"(reference=w465, error in=w464, "dev"=w463) -> ()  [unwired: 2 in, 5 out]
                }
                frame True {
                  n176 = local read "Setup group"() -> (w471:string[][])
                  n177 = for {
                    shift-right: [w476] -> _
                    shift-left: "" -> [w475]
                    tunnel: w471 -> [w477] mode=indexing
                    n178 = Index Array(array=w477, index #1=3 ("index"), index #2=4 ("index"), index #3=5 ("index")) -> (element #1=w484:string, element #2=w476:string, element #3=w479:string)
                    n179 = Decimal String To Number(string=w479) -> (number=w483:i32)  [unwired: 2 in, 1 out]
                    n180 = Not Equal?(x=w476, y=w475) -> (x != y?=w474:bool)
                    n181 = Increment(x=w483) -> (x+1=w473:i32)
                    n182 = case shown="True" w474 {
                      tunnel: w476 -> [_ w491]
                      frame False {
                      }
                      frame True {
                        n183 = call "Connect to Laser_Dx_client.vi"("Laser IP Number"=w491, "error in (no error)"=errorcluster {"status"=FALSE, "code"=0, "source"=""}) -> ("Laser_Dx"=w490:refnum<k7>, "error out"=w489:errorcluster, "Channel"=w488:i64)
                        n184 = invoke class="IBSALaser" method="ShutterClosed"(reference=w490, error in=w489, "dev"=w488) -> ()  [unwired: 2 in, 5 out]
                      }
                    }
                    n185 = call "Connect_to_BSA_F600.vi"("BSA IP Number"=w484) -> ("error out"=w485:errorcluster, "F600"=w486:refnum<k7>)  [unwired: 1 in]
                    n186 = invoke class="IBSA" method="SetBraggCellOutput"(reference=w486, error in=w485, "output"=w473, "activate"=0 ("SetBraggCellOutputFreq")) -> ()  [unwired: 1 in, 5 out]
                  }
                }
              }
            }
          }
          "Error Message" <- w235
          n187 = case shown="False" w238 {
            tunnel: [TRUE ("OK Button") "OK Button"] -> w242
            frame False {
            }
            frame True {
            }
          }
          n188 = Compound Arithmetic op=AND(w237, invert "stop") -> (w236:bool)
          n189 = Select(t=w241, s=w242, f=w240) -> (s? t:f=w239:string)
        }
      }
    }
    frame #4 {
      n190 = case shown="False" w493 {
        tunnel: w494 -> [w496 _]
        tunnel: w492 -> [w495 _]
        frame False {
          w503 = FALSE  # exists?
          n191 = local read "Traverse Control"() -> (w502:T3)
          n192 = Array Size(array=w502) -> (size(s)=w501:i32)
          n193 = local read "Results"() -> (w499:string[][])
          n194 = Number To Decimal String(number=w501) -> (decimal integer string=w500:string)  [unwired: 1 in]
          n195 = call "Beam_Check_Titles.vi"() -> ("Titles"=w497:string[])
          n196 = for {
            tunnel: w500 -> [w512]
            tunnel: w499 -> [w510] mode=indexing
            tunnel: [w513] -> w498 mode=indexing
            tunnel: w496 -> [w511] mode=indexing
            tunnel: w495 -> [w508] mode=indexing
            n197 = Number To Fractional String(number=w508, precision (6)=i16 2) -> (F-format string=w507:string)  [unwired: 2 in]
            n198 = Build Array (concatenate)(w511, w512, w507, w510) -> (w513:string[])
          }
          n199 = global read "Constants_global.vi" "All_Users"() -> (w505:path)
          n200 = Build Path(base path=w505, name or relative path="Beam_Check_Positions.xls" ("Substring")) -> (appended path=w506:path)
          n201 = call "Write_Ch_data_file.vi"("exists?"=w503, "Channel Values"=w498, "Channel names"=w497, "Filename"=w506) -> ()  [unwired: 3 in, 5 out]
        }
        frame True {
        }
      }
    }
  }
